vi "Add Shortcut Menu.vi"(7 "Control":refnum<class "OnShortcutMenuHandler.lvclass">, 8 "error in (no error)":errorcluster, 10 "CtlRef":refnum<vi>, 11 "Control Event Registrations in":refnum<class "Control Event Registrations.lvclass">) -> (0 "error out":errorcluster, 3 "Control Event Registrations out":refnum<class "Control Event Registrations.lvclass">)   [LabVIEW 2020, in "VolatusGUI.lvlib" / "Control Event Registrations.lvclass"]
uses:
  Control Event Registrations.lvclass
  Control Event Registrations.lvclass/Control Event Registrations.ctl
  Control Event.ctl
  VolatusGUI.lvlib
  Event Registration.ctl
  OnShortcutMenuHandler/OnShortcutMenuHandler.lvclass
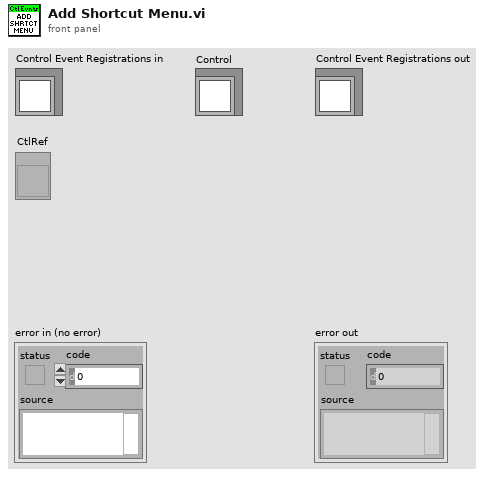
[diagram p1: front panel]
types:
  T1 = typedef "VolatusGUI.lvlib/Event Registration.ctl" = cluster{"CtlRef":refnum<vi>, "Event":T2}
  T2 = typedef "VolatusGUI.lvlib/Control Event.ctl" = enum16{"Value Change", "Shortcut Menu"}
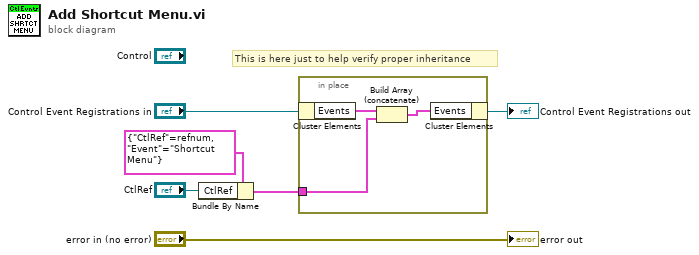
[diagram p0: block diagram]
diagram:
  # "This is here just to help verify proper inheritance"
  n1 = Bundle By Name(cluster=T1 {"CtlRef"=refnum, "Event"=enum."Shortcut Menu"} ("Event Registration"), "CtlRef"="CtlRef") -> (w2:T1)
  n2 = in-place {
    in-place-border: w2 -> [w8]
    n3 = in-place-cluster #1("Control Event Registrations in") -> ("Events"=w9:T1[])
    n4 = Build Array (concatenate)(w9, w8) -> (w7:T1[])
    n5 = in-place-cluster #1("Events"=w7) -> (→"Control Event Registrations out":refnum<class "Control Event Registrations.lvclass">)
  }
  "error out" <- "error in (no error)"
